vi "Event Viewer.vi"(8 "Error in (no error)":errorcluster) -> (0 "Error out":errorcluster)   [LabVIEW 2022 SP3]
uses:
  <vilib>/NI/Event Logger Library/EventLog/Read_TDMS.vi
  <vilib>/NI/Event Logger Library/EventLog/EventLog.lvclass
panel:
  in  "Select a Log":i32(listbox)
  out "Description":string
  in  "Multicolumn Listbox":i32(listbox)=-1
  in  "EventLog File Path":path
  # "Events Viewer"
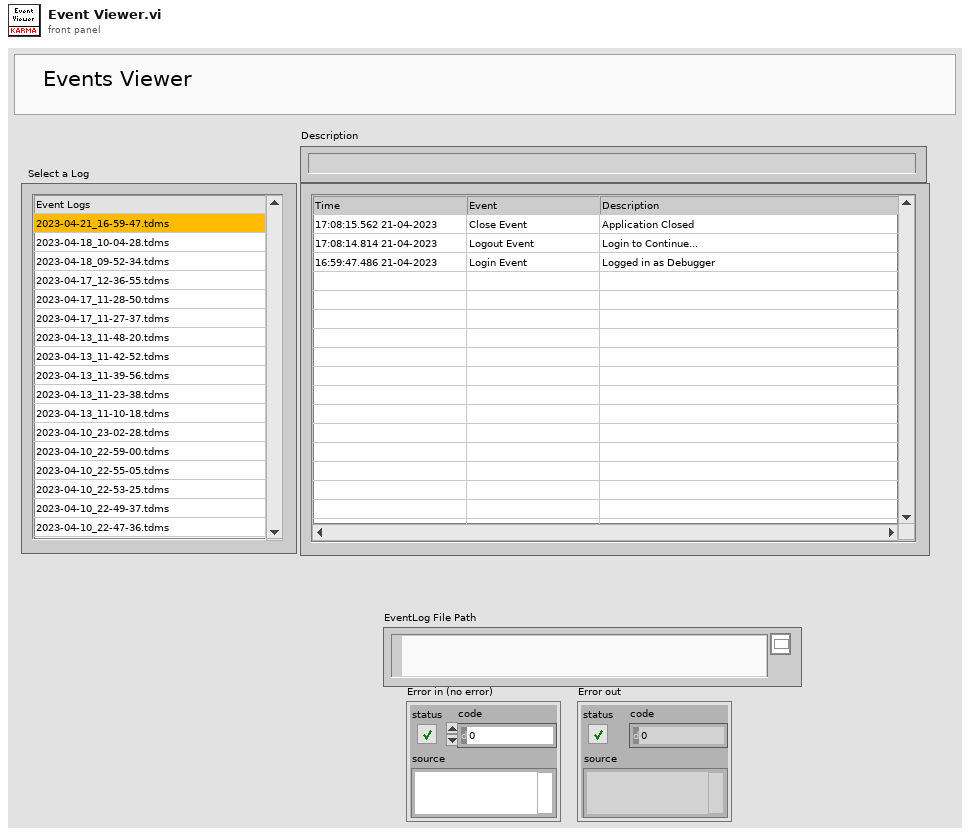
[diagram p1: front panel]
types:
  T1 = enum16{"Poll", "Initialize", "Load File", "Error", "Exit"}
  T2 = typedef "EventBuffer.lvclass/Event_1_0.ctl" = cluster{"TimeStamp":timestamp, "Name":string, "Description":string}
  T3 = typedef "Paths.ctl" = cluster{"Configuration":path, "Event Logs":path, "Error Logs":path, "Configuration.ini":path}
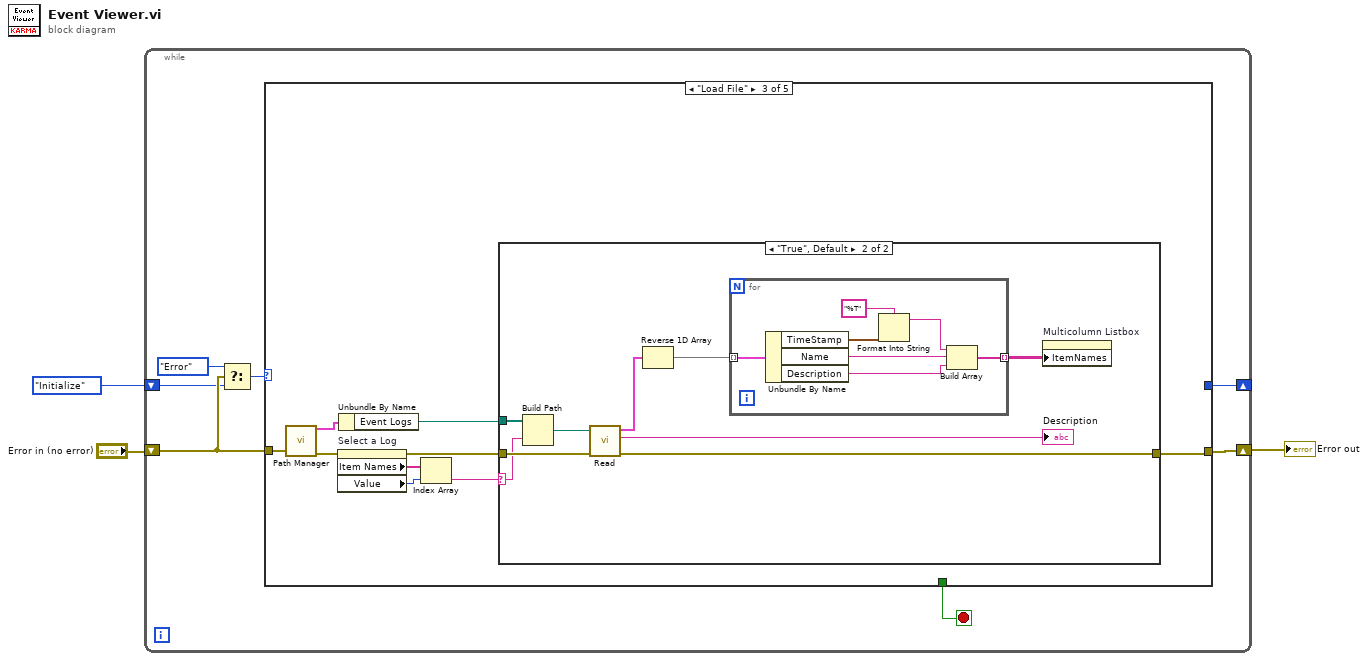
[diagram p0: block diagram]
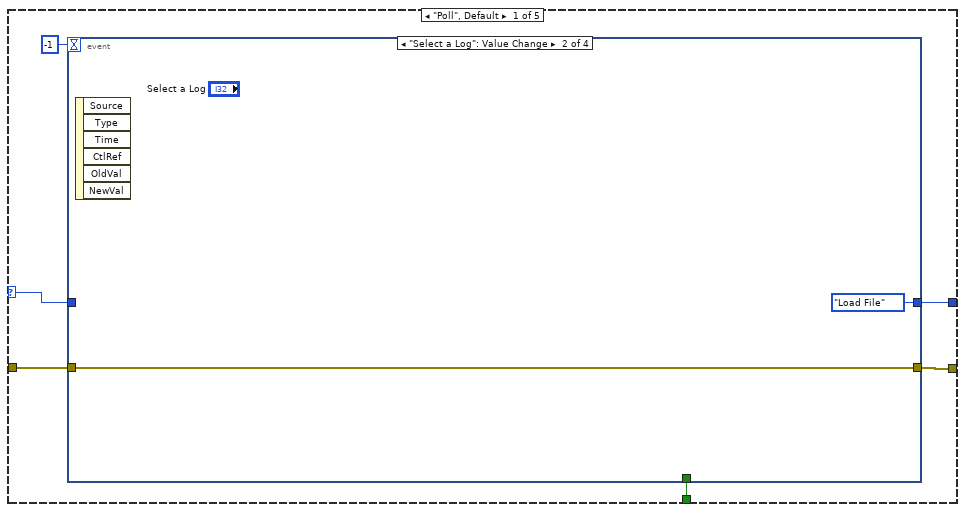
[diagram p2: hidden frame]
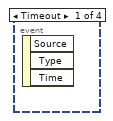
[diagram p3: hidden frame]
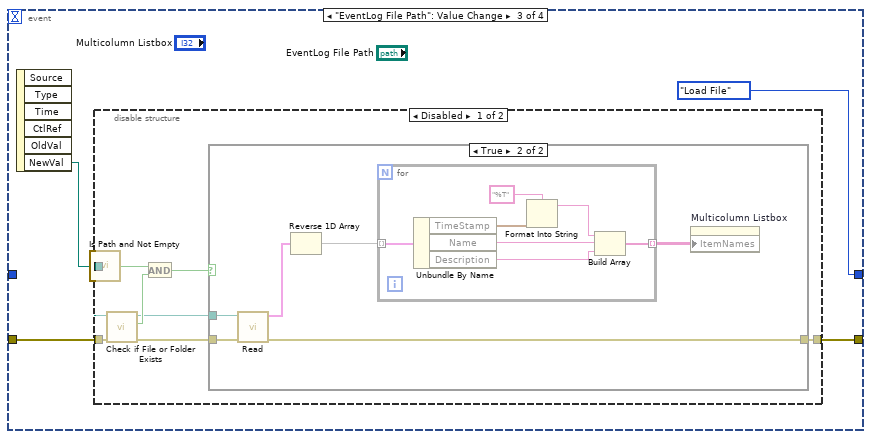
[diagram p4: hidden frame]
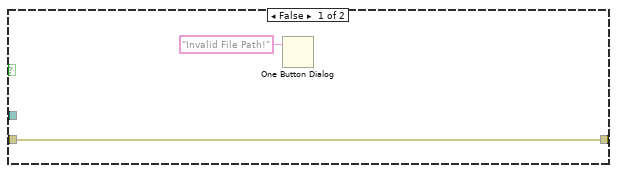
[diagram p5: hidden frame]
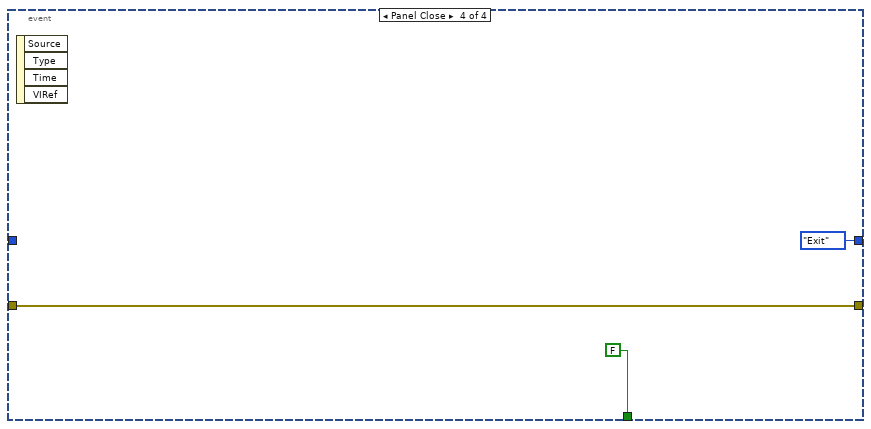
[diagram p7: hidden frame]
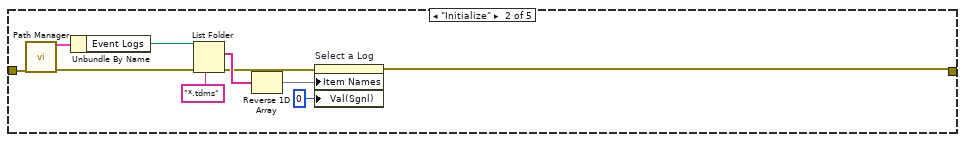
[diagram p8: hidden frame]
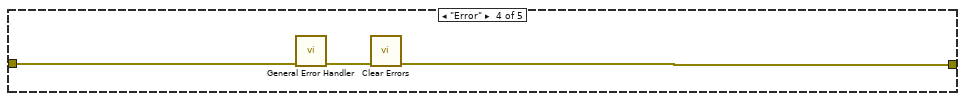
[diagram p10: hidden frame]
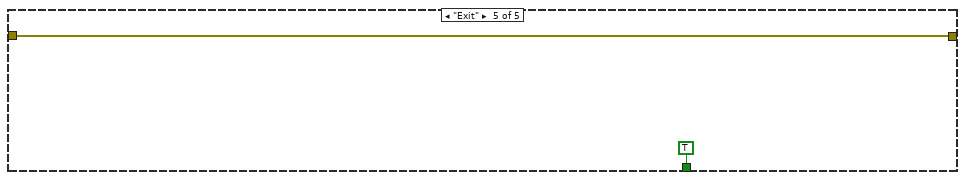
[diagram p11: hidden frame]
diagram:
  n1 = while {
    shift-right: [w8] -> _
    shift-left: T1."Initialize" -> [w6]
    shift-right: [w9] -> w3
    shift-left: "Error in (no error)" -> [w7]
    stop <- w10 stop-if-true
    n2 = Select(t=T1."Error", s=w7, f=w6) -> (s? t:f=w4:T1)
    n3 = case shown="\"Load File\"" w4 {
      selector: w4 -> [w14 _ _ _ _]
      tunnel: [w16 _ _ _ TRUE] -> w10
      tunnel: [w15 w50 w62 w87 w90] -> w9
      tunnel: w7 -> [w12 w51 w67 w86 w90]
      tunnel: [w11 _ _ _ _] -> w8
      frame "Poll", Default {
        n4 = event shown="[1] \"Select a Log\": Value Change" {
          selector: _ -> [_ _ _ _]
          dyn-events: _ -> [_ _ _ _]
          timeout: -1 -> [_ _ _ _]
          tunnel: [_ _ _ FALSE] -> w16
          tunnel: [_ w17 w22 w47] -> w15
          tunnel: w14 -> [_ _ _ _]
          tunnel: w12 -> [_ w17 w20 w47]
          tunnel: [_ T1."Load File" T1."Load File" T1."Exit"] -> w11
          event Timeout {
            n5 = event-data() -> ()  [unwired: 1 in, 3 out]
          }
          event "Select a Log": Value Change {
            n6 = event-data() -> ()  [unwired: 1 in, 6 out]
          }
          event "EventLog File Path": Value Change {
            n7 = event-data() -> ("NewVal"=w21:path)  [unwired: 1 in, 5 out]
            n8 = disable-structure shown="Disabled" {
              disable-tunnel: [w30 w46] -> w22
              disable-tunnel: w21 -> [w28 _]
              disable-tunnel: w20 -> [w23 w46]
              frame Disabled {
                n9 = call <vilib>:"Is Path and Not Empty.vi"("path"=w28) -> ("Is Path and Not Empty?"=w26:bool)  [unwired: 4 in]
                n10 = call <vilib>:"Check if File or Folder Exists.vi"("error in (no error)"=w23, "path"=w28) -> ("error out"=w29:errorcluster, "file or folder exists?"=w25:bool, "dup path"=w24:path)  [unwired: 7 in]
                n11 = And(x=w26, y=w25) -> (x .and. y?=w27:bool)
                n12 = case shown="True" w27 {
                  tunnel: [w32 w35] -> w30
                  tunnel: w29 -> [w32 w34]
                  tunnel: w24 -> [_ w33]
                  frame False {
                    n13 = One Button Dialog(message="Invalid File Path!") -> ()  [unwired: 1 in, 1 out]
                  }
                  frame True {
                    n14 = call-poly <vilib>:"Read.vi"("error in (no error)"=w34, "Path"=w33) -> ("error out"=w35:errorcluster, "Events"=w38:T2[])  [unwired: 6 in, 2 out]
                    n15 = Reverse 1D Array(array=w38) -> (reversed array=w37:T2[])
                    n16 = for {
                      tunnel: w37 -> [w45] mode=indexing
                      tunnel: [w39] -> w36 mode=indexing
                      n17 = Unbundle By Name(w45) -> ("TimeStamp"=w44:timestamp, "Name"=w41:string, "Description"=w40:string)
                      n18 = Format Into String(format string="%T", w44) -> (resulting string=w42:string)  [unwired: 2 in, 1 out]
                      n19 = Build Array(w42, w41, w40) -> (w39:string[])
                    }
                    n20 = property on="Multicolumn Listbox" class="MCListbox (strict)"("ItemNames"=w36) -> ()  [unwired: 2 in, 2 out]
                  }
                }
              }
              frame Enabled {
              }
            }
          }
          event Panel Close {
            n21 = event-data() -> ()  [unwired: 1 in, 4 out]
          }
        }
      }
      frame "Initialize" {
        n22 = call "Path Manager.vi"("error in (no error)"=w51) -> ("Cluster"=w52:T3, "Error out"=w57:errorcluster)  [unwired: 13 in]
        n23 = Unbundle By Name(w52) -> ("Event Logs"=w54:path)
        n24 = List Folder(path=w54, pattern="*.tdms", error in=w57) -> (filenames=w56:string[], error out=w55:errorcluster)  [unwired: 1 in, 2 out]
        n25 = Reverse 1D Array(array=w56) -> (reversed array=w58:string[])
        n26 = property on="Select a Log" class="LstBox (strict)"(error in=w55, "Item Names"=w58, "Val(Sgnl)"=0 ("Value (Signaling)")) -> (error out=w50:errorcluster)  [unwired: 1 in, 1 out]
      }
      frame "Load File" {
        n27 = call "Path Manager.vi"("error in (no error)"=w67) -> ("Cluster"=w68:T3, "Error out"=w63:errorcluster)  [unwired: 13 in]
        n28 = property on="Select a Log" class="LstBox (strict)"(error in=w63) -> (error out=w64:errorcluster, "Item Names"=w66:string[], "Value"=w65:i32)  [unwired: 1 in, 1 out]
        n29 = Unbundle By Name(w68) -> ("Event Logs"=w60:path)
        n30 = Index Array(array=w66, index=w65) -> (element=w61:string)
        n31 = case shown="\"True\", Default" w61 {
          selector: w61 -> [_ w70]
          tunnel: w64 -> [w69 w78]
          tunnel: [w69 w74] -> w62
          tunnel: w60 -> [_ w72]
          frame "" {
          }
          frame "True", Default {
            n32 = Build Path(base path=w72, name or relative path=w70) -> (appended path=w71:path)
            n33 = call-poly <vilib>:"Read.vi"("error in (no error)"=w78, "Path"=w71) -> ("error out"=w74:errorcluster, "Description"=→"Description":string, "Events"=w77:T2[])  [unwired: 6 in, 1 out]
            n34 = Reverse 1D Array(array=w77) -> (reversed array=w76:T2[])
            n35 = for {
              tunnel: w76 -> [w85] mode=indexing
              tunnel: [w79] -> w75 mode=indexing
              n36 = Unbundle By Name(w85) -> ("TimeStamp"=w84:timestamp, "Name"=w81:string, "Description"=w80:string)
              n37 = Format Into String(format string="%T", w84) -> (resulting string=w82:string)  [unwired: 2 in, 1 out]
              n38 = Build Array(w82, w81, w80) -> (w79:string[])
            }
            n39 = property on="Multicolumn Listbox" class="MCListbox (strict)"("ItemNames"=w75) -> ()  [unwired: 2 in, 2 out]
          }
        }
      }
      frame "Error" {
        n40 = call <vilib>:"General Error Handler.vi"("error in (no error)"=w86) -> ("error out"=w88:errorcluster)  [unwired: 10 in, 4 out]
        n41 = call <vilib>:"Clear Errors.vi"("error in (no error)"=w88) -> ("error out"=w87:errorcluster)  [unwired: 5 in, 1 out]
      }
      frame "Exit" {
      }
    }
  }
  "Error out" <- w3
